vi "VR Make Path.vi"(10 "Channel":i32, 11 "Digital in":refnum<vi>) -> (3 "Output path":path)   [LabVIEW 2012]
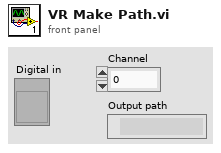
[diagram p1: front panel]
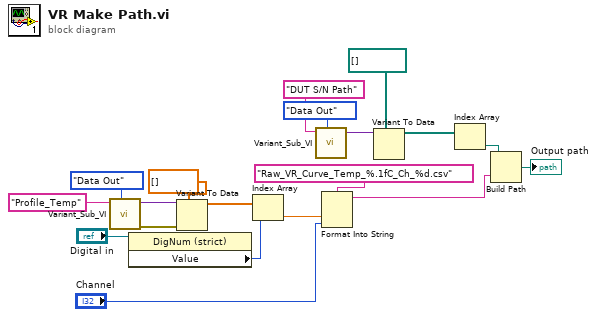
[diagram p0: block diagram]
diagram:
  n1 = call "Variant_Sub_VI.vi"("Mode"=enum16{"Init", "Data In", "Data Out"}."Data Out", "Data Name"="Profile_Temp") -> ("error out"=w6:errorcluster, "Out"=w8:variant)  [unwired: 8 in]
  n2 = property on="Property Node" class="DigNum (strict)"(reference="Digital in") -> ("Value"=w10:i32)  [unwired: 1 in, 2 out]
  n3 = Variant To Data(error in=w6, type=dbl[] [], Variant=w8) -> (data=w4:dbl[])  [unwired: 1 out]
  n4 = Index Array(array=w4, index=w10) -> (element=w12:dbl)
  n5 = call "Variant_Sub_VI.vi"("Mode"=enum16{"Init", "Data In", "Data Out"}."Data Out", "Data Name"="DUT S/N Path") -> ("Out"=w18:variant)  [unwired: 8 in, 1 out]
  n6 = Format Into String(format string="Raw_VR_Curve_Temp_%.1fC_Ch_%d.csv", w12, "Channel") -> (resulting string=w19:string)  [unwired: 2 in, 1 out]
  n7 = Variant To Data(type=path[] [], Variant=w18) -> (data=w15:path[])  [unwired: 1 in, 1 out]
  n8 = Index Array(array=w15) -> (element=w14:path)  [unwired: 1 in]
  n9 = Build Path(base path=w14, name or relative path=w19) -> (appended path=→"Output path":path)
